vi "robotprofile.vi"() -> ()   [LabVIEW 2019]
doc: "This global variable contains bypass information for sensors"
panel:
  out "Enable_Shifting":bool
  out "Pressure_Transducer_Bypass":bool
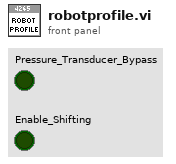
[diagram p1: front panel]
diagram:
